vi "Prog10.vi"() -> ()   [LabVIEW 2021]
panel:
  out "substring 8":string
  out "substring 7":string
  out "substring 6":string
  out "substring 5":string
  out "substring 4":string
  out "substring 3":string
  out "substring 2":string
  out "substring":string
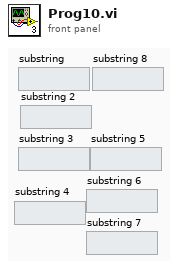
[diagram p1: front panel]
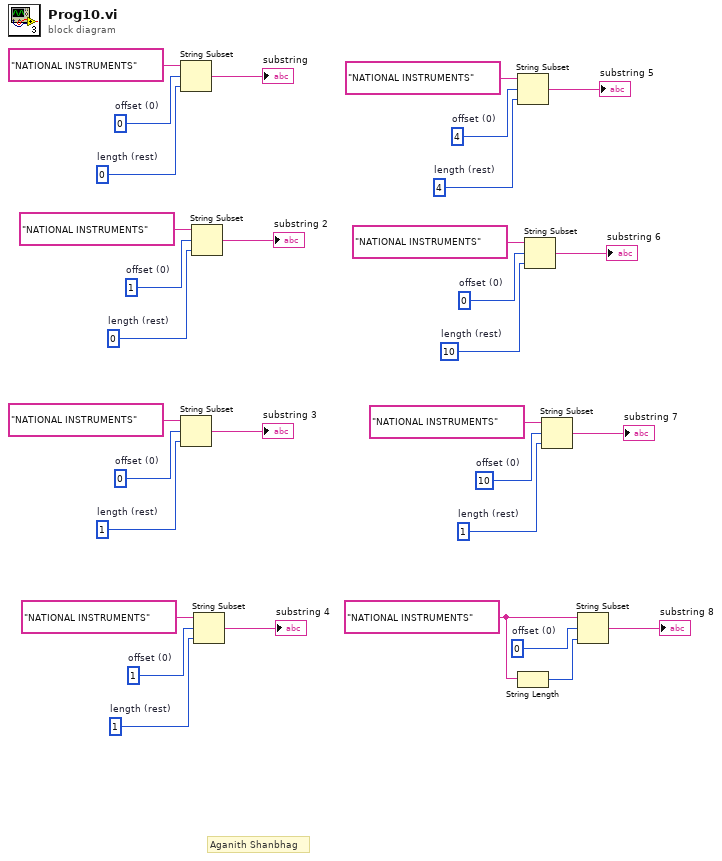
[diagram p0: block diagram]
diagram:
  w4 = 0  # offset (0)
  w2 = "NATIONAL INSTRUMENTS"
  w6 = 1  # length (rest)
  w7 = 10  # offset (0)
  w10 = 10  # length (rest)
  w11 = 0  # offset (0)
  w14 = 4  # length (rest)
  w15 = 4  # offset (0)
  w18 = 1  # length (rest)
  w19 = 1  # offset (0)
  w22 = 1  # length (rest)
  w23 = 0  # offset (0)
  w26 = 0  # length (rest)
  w27 = 1  # offset (0)
  w30 = 0  # length (rest)
  w31 = 0  # offset (0)
  # "Aganith Shanbhag"
  n1 = String Subset(string="NATIONAL INSTRUMENTS", offset (0)=w31, length (rest)=w30) -> (substring=→"substring":string)
  n2 = String Subset(string="NATIONAL INSTRUMENTS", offset (0)=w23, length (rest)=w22) -> (substring=→"substring 3":string)
  n3 = String Subset(string="NATIONAL INSTRUMENTS", offset (0)=w27, length (rest)=w26) -> (substring=→"substring 2":string)
  n4 = String Subset(string="NATIONAL INSTRUMENTS", offset (0)=w19, length (rest)=w18) -> (substring=→"substring 4":string)
  n5 = String Subset(string="NATIONAL INSTRUMENTS", offset (0)=w15, length (rest)=w14) -> (substring=→"substring 5":string)
  n6 = String Length(string=w2) -> (length=w1:i32)
  n7 = String Subset(string="NATIONAL INSTRUMENTS", offset (0)=w11, length (rest)=w10) -> (substring=→"substring 6":string)
  n8 = String Subset(string="NATIONAL INSTRUMENTS", offset (0)=w7, length (rest)=w6) -> (substring=→"substring 7":string)
  n9 = String Subset(string=w2, offset (0)=w4, length (rest)=w1) -> (substring=→"substring 8":string)
